vi "SPI write.vi"(7 "SPI Address":u16, 8 "error in":errorcluster, 9 "Value":bool, 10 "Bit":u16, 11 "FPGA SPI config ref":T1) -> (0 "error out":errorcluster, 3 "FPGA SPI config out":T1)   [LabVIEW 2013]
uses:
  FPGA_spi_config.ctl
  <vilib>/rvi/interface/common/niFpgaWaitOnOcc.vi
  <vilib>/Utility/error.llb/Error Cluster From Error Code.vi
  <vilib>/rvi/errors/niLvFpgaAdjustHostInterfaceError.vi
  <vilib>/rvi/interface/nirviReadWriteControl/nirviReadWriteControl.xnode
  NiFpgaLv.dll
  <vilib>/rvi/interface/Simulation/niFpgaSimulationCallBeginRW.vi
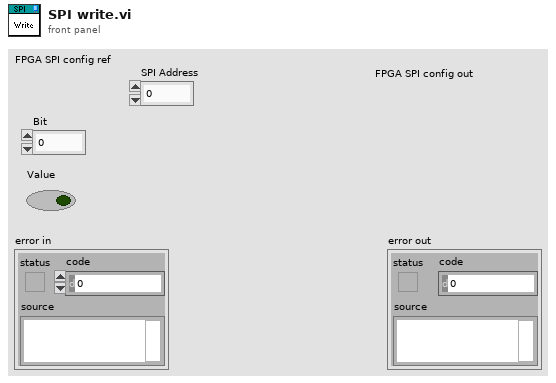
[diagram p1: front panel]
types:
  T1 = typedef "FPGA_spi_config.ctl" = refnum<k20>
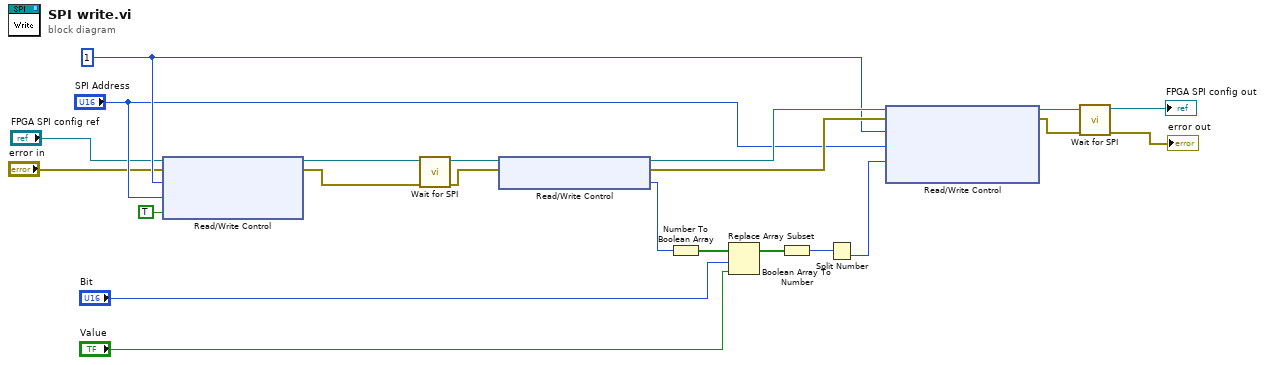
[diagram p0: block diagram]
diagram:
  w6 = u8 1 ("IO Module\\SPI Device")
  n1 = xnode "Read/Write Control"("FPGA VI Reference In"="FPGA SPI config ref", "error in"="error in", "IO Module\\SPI Device"=w6, "IO Module\\SPI Address"="SPI Address", "IO Module\\SPI Read"=TRUE ("IO Module\\SPI Read")) -> ("FPGA VI Reference Out"=w21:T1, "error out"=w20:errorcluster)
  n2 = call "Wait for SPI.vi"("error in"=w20, "FPGA SPI config ref"=w21) -> ("error out"=w18:errorcluster, "FPGA SPI config out"=w19:T1)  [unwired: 7 in, 1 out]
  n3 = xnode "Read/Write Control"("FPGA VI Reference In"=w19, "error in"=w18) -> ("FPGA VI Reference Out"=w10:T1, "error out"=w8:errorcluster, "IO Module\\SPI Read Data"=w12:u8)
  n4 = Number To Boolean Array(number=w12) -> (Boolean array=w17:bool[])
  n5 = Replace Array Subset(array=w17, new element="Value", index="Bit") -> (w16:bool[])
  n6 = Boolean Array To Number(Boolean array=w16) -> (number=w15:u32)
  n7 = Split Number(x=w15) -> (lo(x)=w11:u16)  [unwired: 1 out]
  n8 = xnode "Read/Write Control"("FPGA VI Reference In"=w10, "error in"=w8, "IO Module\\SPI Device"=w6, "IO Module\\SPI Address"="SPI Address", "IO Module\\SPI Write Data"=w11) -> ("FPGA VI Reference Out"=w9:T1, "error out"=w7:errorcluster)  [unwired: 1 in]
  n9 = call "Wait for SPI.vi"("error in"=w7, "FPGA SPI config ref"=w9) -> ("error out"=→"error out":errorcluster, "FPGA SPI config out"=→"FPGA SPI config out":T1)  [unwired: 7 in, 1 out]
